vi "CANopenReadSDO+.vi"(5 "Node ID":u32, 6 "error in":errorcluster, 7 "Sub Index":u8 format="%.0x", 8 "Index":u16=4104 format="%.0x", 9 "FPGA VI Reference In":refnum<k20>) -> (0 "error out":errorcluster, 1 "Data":u8[](array[numeric]), 3 "FPGA VI Reference Out":refnum<k20>, 4 "Data (ASCII)":string)   [LabVIEW 2016]
doc: "This VI Reads incomming SDO messages for single messages as well as for block messages."
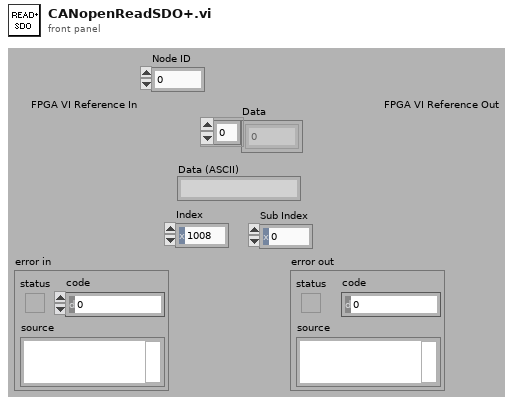
[diagram p1: front panel]
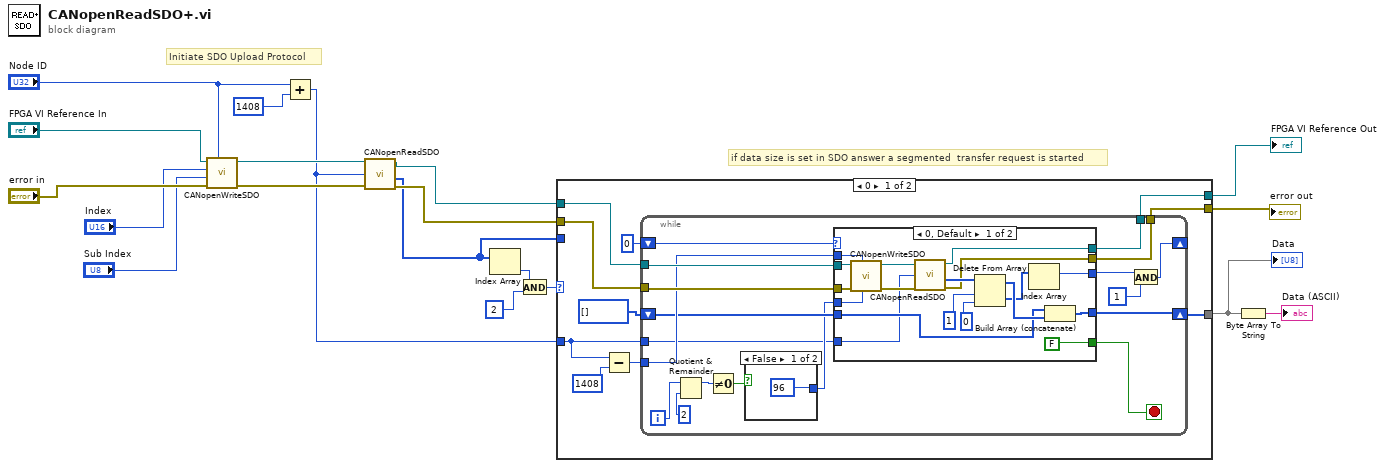
[diagram p0: block diagram]
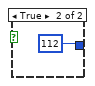
[diagram p2: hidden frame]
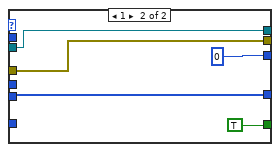
[diagram p3: hidden frame]
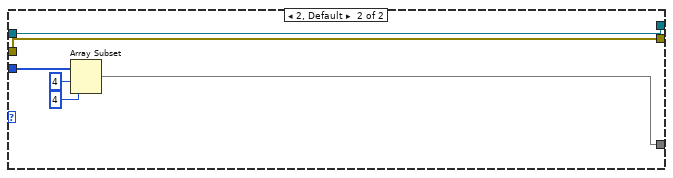
[diagram p4: hidden frame]
diagram:
  # "Initiate SDO Upload Protocol"
  # "if data size is set in SDO answer a segmented  transfer request is started"
  n1 = call "CANopenWriteSDO.vi"("Node ID"="Node ID", "error in"="error in", "Sub Index"="Sub Index", "Index"="Index", "FPGA VI Reference In"="FPGA VI Reference In") -> ("error out"=w4:errorcluster, "FPGA VI Reference Out"=w3:refnum<k20>)  [unwired: 5 in]
  n2 = Add(x="Node ID", y=u32 1408) -> (x+y=w1:u32)
  n3 = call "CANopenReadSDO.vi"("FPGA VI Reference In"=w3, "ID"=w1, "error in"=w4) -> ("FPGA VI Reference Out"=w6:refnum<k20>, "Data"=w2:u8[], "error out"=w5:errorcluster)  [unwired: 1 out]
  n4 = Index Array(array=w2) -> (element=w9:u8)  [unwired: 1 in]
  n5 = And(x=w9, y=u8 2) -> (x .and. y?=w19:u8)
  n6 = case shown="0" w19 {
    tunnel: w1 -> [w20 _]
    tunnel: w5 -> [w28 w75]
    tunnel: w6 -> [w27 w76]
    tunnel: [w24 w73] -> w15
    tunnel: [w22 w76] -> w7
    tunnel: [w21 w75] -> w16
    tunnel: w2 -> [_ w74]
    frame 0 {
      n7 = Subtract(x=w20, y=u32 1408) -> (x-y=w26:u32)
      n8 = while {
        tunnel: w28 -> [w47]
        tunnel: w27 -> [w46]
        tunnel: w26 -> [w45]
        shift-right: [w43] -> w24
        shift-left: u8[] [] ("Data") -> [w44]
        shift-right: [w31] -> _
        shift-left: u8 0 -> [w40]
        tunnel: [w33] -> w22
        tunnel: [w32] -> w21
        tunnel: w20 -> [w30]
        i -> [w38]
        stop <- w39 stop-if-true
        n9 = Quotient & Remainder(x=w38, y=2) -> (x-y*floor(x/y)=w36:i32)  [unwired: 1 out]
        n10 = Not Equal To 0?(x=w36) -> (x != 0?=w35:bool)
        n11 = case shown="False" w35 {
          tunnel: [u8 96 u8 112] -> w34
          frame False {
          }
          frame True {
          }
        }
        n12 = case shown="0, Default" w40 {
          tunnel: w47 -> [w67 w68]
          tunnel: w46 -> [w52 w69]
          tunnel: w45 -> [w66 _]
          tunnel: w44 -> [w60 w70]
          tunnel: [w59 w70] -> w43
          tunnel: [w58 u8 0] -> w42
          tunnel: [FALSE TRUE] -> w39
          tunnel: w34 -> [w53 _]
          tunnel: [w55 w69] -> w33
          tunnel: [w54 w68] -> w32
          tunnel: w30 -> [w50 _]
          frame 0, Default {
            n13 = call "CANopenWriteSDO.vi"("Byte0 (h40)"=w53, "Node ID"=w66, "error in"=w67, "FPGA VI Reference In"=w52) -> ("error out"=w65:errorcluster, "FPGA VI Reference Out"=w51:refnum<k20>)  [unwired: 6 in]
            n14 = call "CANopenReadSDO.vi"("FPGA VI Reference In"=w51, "ID"=w50, "error in"=w65) -> ("FPGA VI Reference Out"=w55:refnum<k20>, "Data"=w64:u8[], "error out"=w54:errorcluster)  [unwired: 1 out]
            n15 = Delete From Array(array=w64, length=1, index=0) -> (deleted portion=w57:u8[], array with subset deleted=w61:u8[])
            n16 = Index Array(array=w57) -> (element=w58:u8)  [unwired: 1 in]
            n17 = Build Array (concatenate)(w60, w61) -> (w59:u8[])
          }
          frame 1 {
          }
        }
        n18 = And(x=w42, y=u8 1) -> (x .and. y?=w31:u8)
      }
    }
    frame 2, Default {
      n19 = Array Subset(array=w74, index=4, length=4) -> (w73:u8[])
    }
  }
  "error out" <- w16
  "Data" <- w15
  "FPGA VI Reference Out" <- w7
  n20 = Byte Array To String(unsigned byte array=w15) -> (string=→"Data (ASCII)":string)
